vi "CTRE_ServoBlock_SmartTankStraight.vi"(10 "Timeout (s)":dbl, 11 "Sensored Tank Servo Straight":T9) -> (3 "Sensored Tank":T1={"Sensored Gearbox Left"={"Smart Motor Controller"={"DeviceStatus"={"status"=FALSE, "code"=0, "source"=""}, "Type"=enum."PWM", "PWM"={"PWM Channel"=enum."PWM 1", "DeadBand"={"Name"="", "maxPositivePwm"=0, "minPositivePwm"=0, "centerPwm"=0, "maxNegativePwm"=0, "minNegativePwm"=0, "angularRange"=0}}, "CAN"={"Device Number"=0, "SetOutput VI Ref"=variant(enum8{"Percent VBus", "Current", "Speed", "Position", "Voltage"} enum."Percent VBus"), "GetOutput VI Ref"=variant(refnum<k1> refnum), "Enable VI Ref"=variant(dbl 12.0), "Disable VI Ref"=variant(enum8{"Percent VBus", "Speed", "Position", "Slave", "Unchanged / Invalid", "Voltage Compensation", "Current", "Motion Profile"} enum."Percent VBus"), "Data"=variant}, "Invert"=FALSE}, "Invert"=FALSE, "Gear Ratio"=0.0}, "Sensored Gearbox Right "={"Smart Motor Controller"={"DeviceStatus"={"status"=FALSE, "code"=0, "source"=""}, "Type"=enum."PWM", "PWM"={"PWM Channel"=enum."PWM 1", "DeadBand"={"Name"="", "maxPositivePwm"=0, "minPositivePwm"=0, "centerPwm"=0, "maxNegativePwm"=0, "minNegativePwm"=0, "angularRange"=0}}, "CAN"={"Device Number"=0, "SetOutput VI Ref"=variant(enum8{"Percent VBus", "Current", "Speed", "Position", "Voltage"} enum."Percent VBus"), "GetOutput VI Ref"=variant(refnum<k1> refnum), "Enable VI Ref"=variant(dbl 12.0), "Disable VI Ref"=variant(enum8{"Percent VBus", "Speed", "Position", "Slave", "Unchanged / Invalid", "Voltage Compensation", "Current", "Motion Profile"} enum."Percent VBus"), "Data"=variant}, "Invert"=FALSE}, "Invert"=FALSE, "Gear Ratio"=0.0}, "Wheel Radius"=0.0, "Distance Between Wheels"=0.0})   [LabVIEW 2016]
uses:
  <vilib>/Rock Robotics/WPI/ThirdParty/CanMotor/CTRLib-LV-TalonSRX/Framework/SensoredTank.ctl
  <vilib>/Rock Robotics/WPI/ThirdParty/CanMotor/CTRLib-LV-TalonSRX/Framework/SensoredGearbox.ctl
  <vilib>/Rock Robotics/WPI/MotorControl/WPI_MotorControlDeviceRef.ctl
  <vilib>/Rock Robotics/WPI/MotorControl/WPI_MotorControlType.ctl
  <vilib>/Rock Robotics/SystemInterfaces/DIO/FPGA_DIOPWMChannel.ctl
  <vilib>/Rock Robotics/WPI/PWM/WPI_PWMDeadband.ctl
  <vilib>/Rock Robotics/WPI/ThirdParty/CanMotor/CTRLib-LV-TalonSRX/CTRE_CANTalonSRX_ControlMode.ctl
  <vilib>/Rock Robotics/WPI/ThirdParty/CanMotor/CTRLib-LV-TalonSRX/Framework/ServoParams.ctl
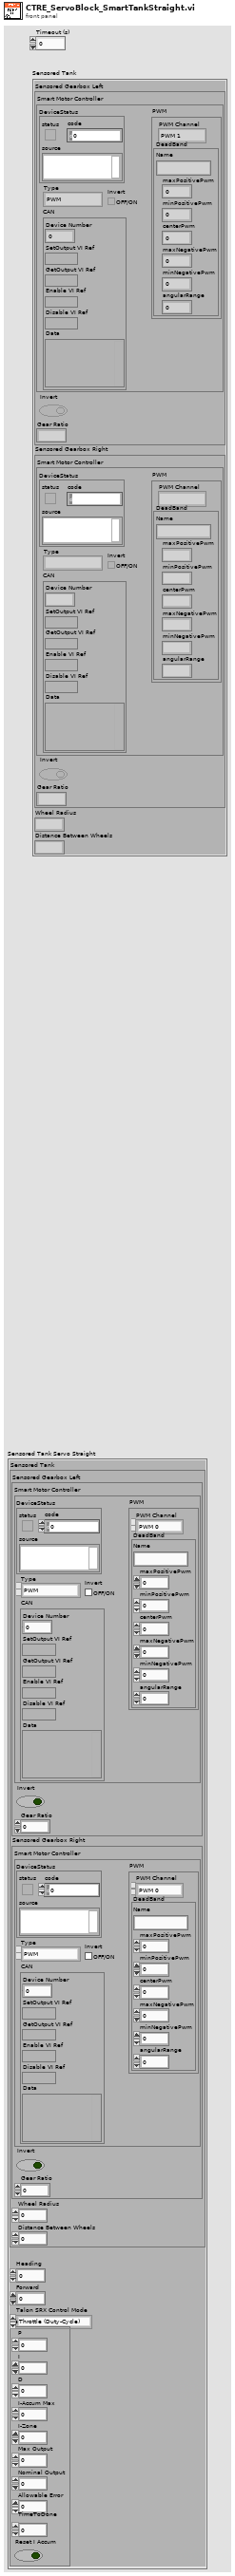
[diagram p1: front panel]
types:
  T1 = typedef "SensoredTank.ctl" = cluster{"Sensored Gearbox Left":T2, "Sensored Gearbox Right ":T2, "Wheel Radius":dbl, "Distance Between Wheels":dbl}
  T2 = typedef "SensoredGearbox.ctl" = cluster{"Smart Motor Controller":T3, "Invert":bool, "Gear Ratio":dbl}
  T3 = typedef "WPI_MotorControlDeviceRef.ctl" = cluster{"DeviceStatus":errorcluster, "Type":T4, "PWM":cluster{"PWM Channel":T5, "DeadBand":T6}, "CAN":cluster{"Device Number":u8, "SetOutput VI Ref":variant, "GetOutput VI Ref":variant, "Enable VI Ref":variant, "Disable VI Ref":variant, "Data":variant}, "Invert":bool}
  T4 = typedef "WPI_MotorControlType.ctl" = enum16{"PWM", "CAN"}
  T5 = typedef "FPGA_DIOPWMChannel.ctl" = enum8{"PWM 0", "PWM 1", "PWM 2", "PWM 3", "PWM 4", "PWM 5", "PWM 6", "PWM 7", "PWM 8", "PWM 9", "PWM MXP 0", "PWM MXP 1", "PWM MXP 2", "PWM MXP 3", "PWM MXP 4", "PWM MXP 5", "PWM MXP 6", "PWM MXP 7", "PWM MXP 8", "PWM MXP 9", "Invalid"}
  T6 = typedef "WPI_PWMDeadband.ctl" = cluster{"Name":string, "maxPositivePwm":i32, "minPositivePwm":i32, "centerPwm":i32, "maxNegativePwm":i32, "minNegativePwm":i32, "angularRange":u16}
  T7 = typedef "CTRE_CANTalonSRX_ControlMode.ctl" = enum16{"Throttle (Duty-Cycle)", "Position Closed-Loop", "Velocity Closed-Loop", "Current Closed-Loop", "Voltage Compensation", "Slave Follower", "Motion Profile", "Motion Magic"}
  T8 = typedef "ServoParams.ctl" = cluster{"P":dbl, "I":dbl, "D":dbl, "I-Accum Max":dbl, "I-Zone":dbl, "Max Output":dbl, "Nominal Output":dbl, "Allowable Error":dbl, "TimeToDone":dbl, "Reset I Accum":bool}
  T9 = cluster{"Sensored Tank":T1, "Heading":dbl, "Forward":dbl, "Talon SRX Control Mode":T7, "Servo Params":T8}
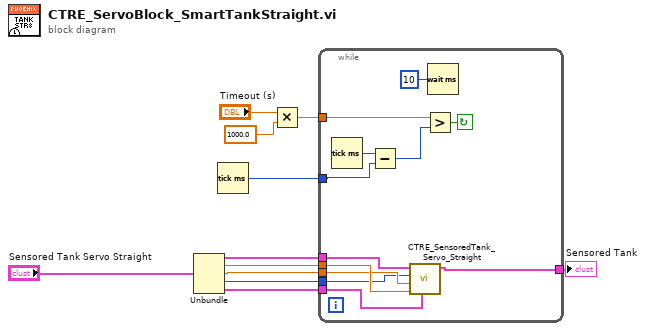
[diagram p0: block diagram]
diagram:
  n1 = Unbundle("Sensored Tank Servo Straight") -> ("Sensored Tank"=w7:T1, "Heading"=w6:dbl, "Forward"=w5:dbl, "Talon SRX Control Mode"=w4:T7, "Servo Params"=w3:T8)
  n2 = Tick Count (ms)() -> (millisecond timer value=w8:u32)
  n3 = Multiply(x="Timeout (s)", y=1000.0 ("Timeout")) -> (x*y=w9:dbl)
  n4 = while {
    tunnel: w9 -> [w21]
    tunnel: w8 -> [w22]
    tunnel: w7 -> [w17]
    tunnel: w6 -> [w16]
    tunnel: w5 -> [w15]
    tunnel: w4 -> [w14]
    tunnel: w3 -> [w13]
    tunnel: [w12] -> w2
    stop <- w20 continue-if-true
    n5 = Tick Count (ms)() -> (millisecond timer value=w23:u32)
    n6 = Subtract(x=w23, y=w22) -> (x-y=w19:u32)
    n7 = call <vilib>:"CTRE_SensoredTank_Servo_Straight.vi"("Servo Params"=w13, "Heading"=w16, "Forward"=w15, "Talon SRX Control Mode"=w14, "Sensored Tank"=w17) -> ("Sensored Tank"=w12:T1)  [unwired: 4 in, 2 out]
    n8 = Greater?(x=w21, y=w19) -> (0:w20:bool)
    n9 = Wait (ms)(milliseconds to wait=u32 10) -> ()  [unwired: 1 out]
  }
  "Sensored Tank" <- w2
